vi "Answer.vi"(10 "Data":string, 11 "CMD 2":T1) -> (1 "dec":u8[](array[numeric]), 2 "Boolean array":bool[][](array[boolean]))   [LabVIEW 2019]
uses:
  FINS/FINS CMD.ctl
  FINS/FINS TCP.lvlib
panel:
  out "data":u16
  out "size":i32
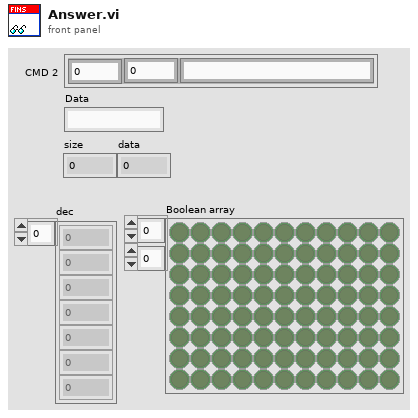
[diagram p1: front panel]
types:
  T1 = typedef "FINS TCP.lvlib/FINS CMD.ctl" = cluster{"MR":u8, "SR":u8, "name":string}
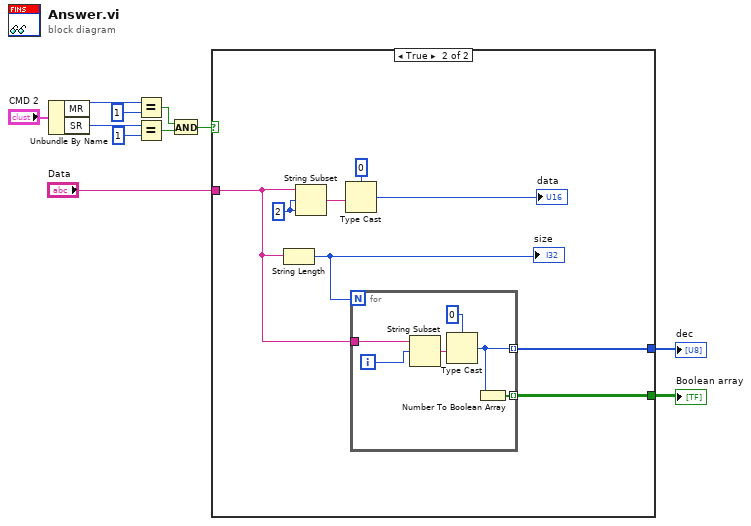
[diagram p0: block diagram]
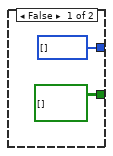
[diagram p2: hidden frame]
diagram:
  n1 = Unbundle By Name("CMD 2") -> ("MR"=w9:u8, "SR"=w8:u8)
  n2 = Equal?(x=w9, y=u8 1) -> (x = y?=w3:bool)
  n3 = Equal?(x=w8, y=u8 1) -> (x = y?=w2:bool)
  n4 = And(x=w3, y=w2) -> (x .and. y?=w1:bool)
  n5 = case shown="True" w1 {
    tunnel: "Data" -> [_ w16]
    tunnel: [bool[][] [] ("Boolean array") w15] -> w5
    tunnel: [u8[] [] w14] -> w4
    frame False {
    }
    frame True {
      w18 = 2 ("length (rest)")
      n6 = String Length(string=w16) -> (length=w17:i32)
      "size" <- w17
      n7 = String Subset(string=w16, offset (0)=w18, length (rest)=w18) -> (substring=w20:string)
      n8 = Type Cast(type=u16 0 ("length (rest)"), x=w20) -> (*(type *) &x=→"data":u16)
      n9 = for {
        N: w17 -> [_]
        tunnel: w16 -> [w27]
        tunnel: [w23] -> w14 mode=indexing
        tunnel: [w22] -> w15 mode=indexing
        i -> [w26]
        n10 = String Subset(string=w27, offset (0)=w26) -> (substring=w24:string)  [unwired: 1 in]
        n11 = Type Cast(type=u8 0 ("length (rest)"), x=w24) -> (*(type *) &x=w23:u8)
        n12 = Number To Boolean Array(number=w23) -> (Boolean array=w22:bool[])
      }
    }
  }
  "dec" <- w4
  "Boolean array" <- w5
